vi "PH_BeamlineInformation.calc Efficiency.vi"(0 "i ref in":refnum<vi>, 5 "error IO":errorcluster) -> (14 "i ref out":refnum<vi>, 19 "error out":errorcluster)   [LabVIEW 2014, in "PH_BeamlineInformation.lvlib"]
doc: "This VI calculates the efficiency (gain and losses) of beamline elements."
uses:
  PH_BeamlineInformation.lvlib
  PH_Beamline_Chief/PH_Beamline_Chief.Section.ctl
  PH_Basics/PH_Common/PH_Common.lvlib
  PH_Beamline_Chief/PH_Beamline_Chief.lvlib
  PH_Basics/PH_SystemInformation/PH_SystemInformation.lvlib
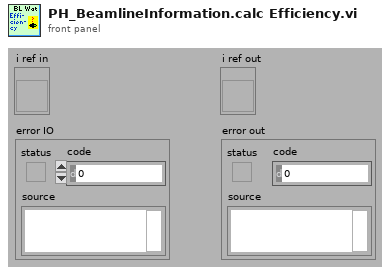
[diagram p1: front panel]
types:
  T1 = typedef "PH_Beamline_Chief.lvlib/PH_Beamline_Chief.Section.ctl" = enum16{"None", "YLF", "fs", "fs-YLF", "ns", "PA-Input", "PA-Undelay", "PA-Delay", "PA-before-Bypass", "PA", "PA-Bypass", "PA-Exit", "PA-LL", "LL", "PA-MA", "MA-Exit", "MA-Z6", "Z6", "MA-LB", "LB-TB2", "LB-TB3"}
  T2 = typedef "PH_BeamlineInformation.lvlib/PH_BeamlineInformation.i attribute.ctl" = cluster{"BL GUI Elements of Services":cluster{"Service Name":string, "GUI Elements":refnum<vi>[], "Status":i32}[], "Powermeters":T3, "Efficiency":T4, "Heads":T5[]}
  T3 = typedef "PH_BeamlineInformation.lvlib/PH_BeamlineInformation.Powermeter.ctl" = cluster{"ns FE":cluster{"GUI Ref":refnum<vi>, "Value":dbl}, "fs FE":cluster{"GUI Ref":refnum<vi>, "Value":dbl}, "PA":cluster{"GUI Ref":refnum<vi>, "Value":dbl}, "MA":cluster{"GUI Ref":refnum<vi>, "Value":dbl}, "Z6 green":cluster{"GUI Ref":refnum<vi>, "Value":dbl}, "Z6 IR":cluster{"GUI Ref":refnum<vi>, "Value":dbl}, "Z6 COS":cluster{"GUI Ref":refnum<vi>, "Value":dbl}}
  T4 = typedef "PH_BeamlineInformation.lvlib/PH_BeamlineInformation.Efficiency.ctl" = cluster{"PA Gain":cluster{"GUI Ref":refnum<vi>, "Value":dbl}, "MA Gain":cluster{"GUI Ref":refnum<vi>, "Value":dbl}, "Z6 green Conversion":cluster{"GUI Ref":refnum<vi>, "Value":dbl}, "Z6 Comp Losses":cluster{"GUI Ref":refnum<vi>, "Value":dbl}}
  T5 = typedef "PH_BeamlineInformation.lvlib/PH_BeamlineInformation.Head.ctl" = cluster{"PowerUnit":T6, "in use":cluster{"Value":bool, "GUI Ref":refnum<vi>, "linked":bool}, "voltage":cluster{"Value":dbl, "GUI Ref":refnum<vi>, "linked":bool}}
  T6 = typedef "PH_PP_Common.lvlib/PH_PP_Common.PUs.ctl" = enum16{"no Info", "PA-19mm-1", "PA-19mm-2", "PA-45mm-PILC", "PA-45mm-MAIN", "MA-PU-1", "MA-PU-2", "MA-PU-3", "MA-PU-4", "MA-PU-5", "MA-PU-6", "MA-FR", "MA-PILC", "PA-45mm-DP"}
  T7 = cluster{"[0]":cluster{"GUI Ref":refnum<vi>, "Value":dbl}, "[1]":cluster{"GUI Ref":refnum<vi>, "Value":dbl}, "[2]":cluster{"GUI Ref":refnum<vi>, "Value":dbl}, "[3]":cluster{"GUI Ref":refnum<vi>, "Value":dbl}}
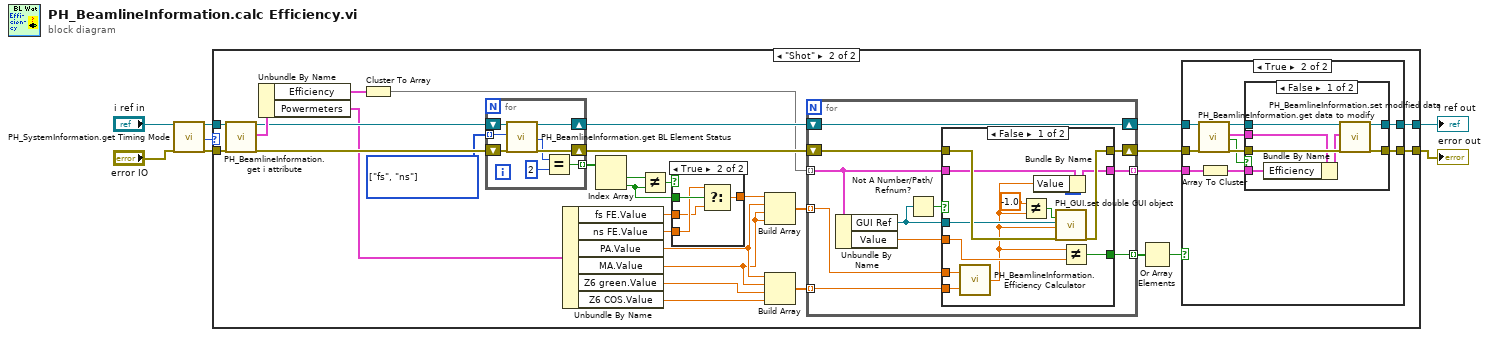
[diagram p0: block diagram]
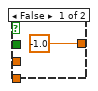
[diagram p5: hidden frame]
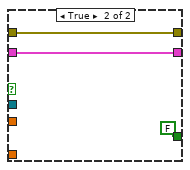
[diagram p6: hidden frame]
diagram:
  n1 = call "PH_SystemInformation.get Timing Mode.vi"("i ref in"="i ref in", "error in (no error)"="error IO") -> ("i ref out"=w2:refnum<vi>, "PHELIX Timing Mode"=w1:enum32{"10 Hz", "0.5 Hz", "Shot"}, "error out"=w4:errorcluster)  [unwired: 15 in]
  n2 = case shown="\"Shot\"" w1 {
    tunnel: [w9 w32] -> w6
    tunnel: [w8 w30] -> w5
    tunnel: w4 -> [w8 w11]
    tunnel: w2 -> [w9 w10]
    frame Default {
    }
    frame "Shot" {
      w34 = T1[] [enum."fs", enum."ns"] items=["None", "YLF", "fs", "fs-YLF", "ns", "PA-Input", "PA-Undelay", "PA-Delay", "PA-before-Bypass", "PA", "PA-Bypass", "PA-Exit", "PA-LL", "LL", "PA-MA", "MA-Exit", "MA-Z6", "Z6", "MA-LB", "LB-TB2", "LB-TB3"]
      n3 = call "PH_BeamlineInformation.get i attribute.vi"("i ref in"=w10, "error in (no error)"=w11) -> ("i ref out"=w39:refnum<vi>, "i attribute"=w40:T2, "error out"=w37:errorcluster)  [unwired: 15 in]
      n4 = Unbundle By Name(w40) -> ("Efficiency"=w19:T4, "Powermeters"=w23:T3)
      n5 = Cluster To Array(cluster=w19) -> (array=w12:cluster{"GUI Ref":refnum<vi>, "Value":dbl}[])
      n6 = for {
        shift-right: [w72] -> w38
        shift-left: w39 -> [w74]
        shift-right: [w71] -> w36
        shift-left: w37 -> [w73]
        tunnel: w34 -> [w68] mode=indexing
        tunnel: [w67] -> w35 mode=indexing
        n7 = call "PH_BeamlineInformation.get BL Element Status.vi"("VI in"=w74, "Beamline Element"=w68, "error in (no error)"=w73) -> ("VI out"=w72:refnum<vi>, "Status"=w69:i32, "error out"=w71:errorcluster)  [unwired: 14 in]
        n8 = Equal?(x=w69, y=2) -> (x = y?=w67:bool)
      }
      n9 = Unbundle By Name(w23) -> ("fs FE.Value"=w22:dbl, "ns FE.Value"=w21:dbl, "PA.Value"=w17:dbl, "MA.Value"=w16:dbl, "Z6 green.Value"=w15:dbl, "Z6 COS.Value"=w14:dbl)
      n10 = Index Array(array=w35) -> (element #1=w25:bool, element #2=w24:bool)  [unwired: 2 in]
      n11 = Not Equal?(x=w25, y=w24) -> (x != y?=w26:bool)
      n12 = case shown="True" w26 {
        tunnel: w24 -> [_ w66]
        tunnel: w21 -> [_ w65]
        tunnel: w22 -> [_ w64]
        tunnel: [-1.0 w63] -> w33
        frame False {
        }
        frame True {
          n13 = Select(t=w65, s=w66, f=w64) -> (s? t:f=w63:dbl)
        }
      }
      n14 = Build Array(w33, w17, w16, w16) -> (w18:dbl[])
      n15 = Build Array(w17, w16, w15, w14) -> (w13:dbl[])
      n16 = for {
        tunnel: w12 -> [w80] mode=indexing
        shift-right: [w85] -> w31
        shift-left: w36 -> [w84]
        shift-right: [w83] -> w29
        shift-left: w38 -> [w83]
        tunnel: [w82] -> w28 mode=indexing
        tunnel: [w79] -> w20 mode=indexing
        tunnel: w18 -> [w78] mode=indexing
        tunnel: w13 -> [w77] mode=indexing
        n17 = Unbundle By Name(w80) -> ("GUI Ref"=w75:refnum<vi>, "Value"=w81:dbl)
        n18 = Not A Number/Path/Refnum?(number/path/refnum=w75) -> (NaN/Path/Refnum?=w76:bool)
        n19 = case shown="False" w76 {
          tunnel: [w97 w99] -> w85
          tunnel: w84 -> [w96 w99]
          tunnel: w75 -> [w95 _]
          tunnel: [w94 FALSE] -> w82
          tunnel: w81 -> [w93 _]
          tunnel: w80 -> [w92 w100]
          tunnel: [w91 w100] -> w79
          tunnel: w78 -> [w90 _]
          tunnel: w77 -> [w89 _]
          frame False {
            n20 = call "PH_BeamlineInformation.Efficiency Calculator.vi"("Later Subystem"=w89, "Former Subsystem"=w90) -> ("Efficiency Factor"=w87:dbl)
            n21 = Not Equal?(x=-1.0, y=w87) -> (x != y?=w88:bool)
            n22 = Bundle By Name(cluster=w92, "Value"=w87) -> (w91:cluster{"GUI Ref":refnum<vi>, "Value":dbl})
            n23 = call "PH_GUI.set double GUI object.vi"("visible (true)"=w88, "GUI object Ref"=w95, "value"=w87, "error in (no error)"=w96) -> ("error out"=w97:errorcluster)  [unwired: 15 in]
            n24 = Not Equal?(x=w87, y=w93) -> (x != y?=w94:bool)
          }
          frame True {
          }
        }
      }
      n25 = Or Array Elements(Boolean array=w28) -> (logical OR=w27:bool)
      n26 = case shown="True" w27 {
        tunnel: [w42 w52] -> w32
        tunnel: w31 -> [w41 w51]
        tunnel: [w41 w50] -> w30
        tunnel: w29 -> [w42 w48]
        tunnel: w20 -> [_ w44]
        frame False {
        }
        frame True {
          n27 = call "PH_BeamlineInformation.get data to modify.vi"("i ref in"=w48, "error in (no error)"=w51) -> ("i ref out"=w47:refnum<vi>, "i attribute"=w45:T2, "timed out"=w46:bool, "error out"=w49:errorcluster)  [unwired: 14 in]
          n28 = Array To Cluster(array=w44) -> (cluster=w43:T7)
          n29 = case shown="False" w46 {
            tunnel: [w59 w61] -> w52
            tunnel: [w58 w60] -> w50
            tunnel: w49 -> [w57 w60]
            tunnel: w47 -> [w56 w61]
            tunnel: w45 -> [w54 _]
            tunnel: w43 -> [w53 _]
            frame False {
              n30 = Bundle By Name(cluster=w54, "Efficiency"=w53) -> (w55:T2)
              n31 = call "PH_BeamlineInformation.set modified data.vi"("i ref in"=w56, "i attribute"=w55, "error in (no error)"=w57) -> ("i ref out"=w59:refnum<vi>, "error out"=w58:errorcluster)  [unwired: 15 in]
            }
            frame True {
            }
          }
        }
      }
    }
  }
  "i ref out" <- w6
  "error out" <- w5
